vi "Error_to_String_Converter.vi"(8 "error in":errorcluster) -> (0 "error out":errorcluster, 3 "String":string)   [LabVIEW 2015]
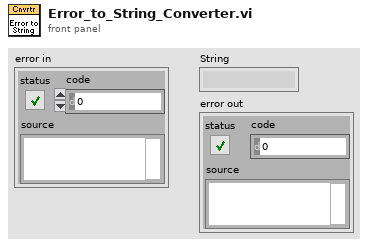
[diagram p1: front panel]
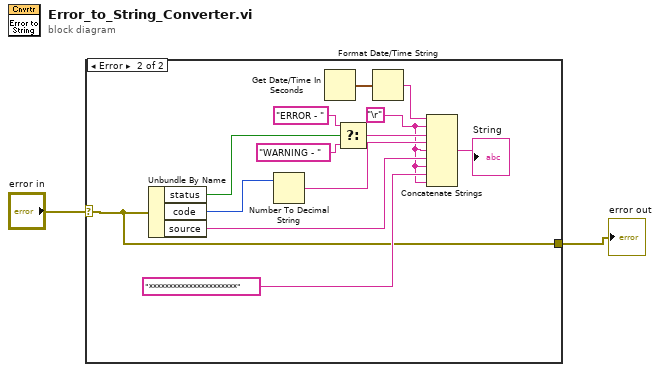
[diagram p0: block diagram]
diagram:
  n1 = case shown="Error" "error in" {
    selector: "error in" -> [w3 w4]
    tunnel: [w3 w4] -> w1
    frame No Error {
    }
    frame Error {
      w5 = "\r"
      n2 = Unbundle By Name(w4) -> ("status"=w13:bool, "code"=w9:i32, "source"=w7:string)
      n3 = Number To Decimal String(number=w9) -> (decimal integer string=w8:string)  [unwired: 1 in]
      n4 = Get Date/Time In Seconds() -> (seconds since 1Jan1904=w14:timestamp)
      n5 = Select(t="ERROR - ", s=w13, f="WARNING - ") -> (s? t:f=w12:string)
      n6 = Format Date/Time String(seconds (now)=w14) -> (date/time string=w15:string)  [unwired: 2 in]
      n7 = Concatenate Strings(w15, w5, w12, w8, w5, w7, w5, "**********************", w5) -> (→"String":string)
    }
  }
  "error out" <- w1
